vi "Export_mapFileName.vi"(1 "MapFunctionStr":string, 2 "Spectrum":refnum<vi>, 3 "SourceFile":path) -> (0 "Dateipfad":path)   [LabVIEW 2010]
panel:
  in  "Dateiendung":string="tsv"
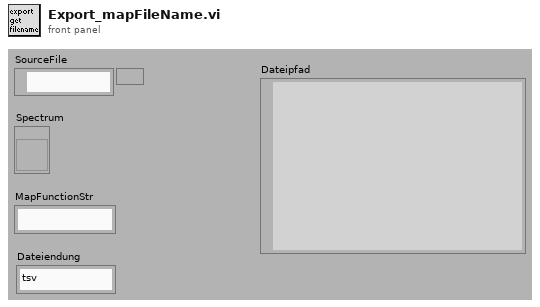
[diagram p1: front panel]
types:
  T1 = typedef "LVCursorListTypeDef.ctl" = cluster{"Name":string, "Color":u32, "Style":u8, "Point Style":u8, "Name Visible":bool, "Allow Drag":bool, "Cursor Mode":u32, "Plot":i32, "Index":i32, "Position":cluster{"X":dbl, "Y":dbl}, "X Scale":u32, "Y Scale":u32, "Watch Plots":i32[], "Watch All Plots":bool, "Plot Area":i32, "Label Offset":cluster{"X":dbl, "Y":dbl}}[]
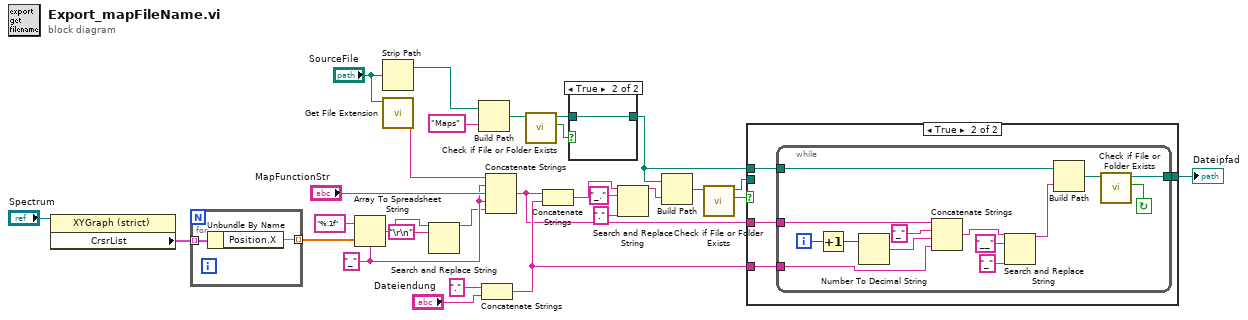
[diagram p0: block diagram]
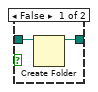
[diagram p2: hidden frame]
diagram:
  w14 = "_" ("String")
  n1 = property on="Eigenschaftsknoten" class="XYGraph (strict)"(reference="Spectrum") -> ("CrsrList"=w20:T1)  [unwired: 1 in, 2 out]
  n2 = for {
    tunnel: w20 -> [w31] mode=indexing
    tunnel: [w30] -> w15 mode=indexing
    n3 = Unbundle By Name(w31) -> ("Position.X"=w30:dbl)
  }
  n4 = Array To Spreadsheet String(delimiter (Tab)=w14, array=w15, 3:"%.1f" ("Format-String")) -> (spreadsheet string=w2:string)
  n5 = Strip Path(path="SourceFile") -> (stripped path=w18:path)  [unwired: 1 out]
  n6 = call <vilib>:"Get File Extension.vi"("file"="SourceFile") -> ("filename without extension"=w17:string)  [unwired: 7 in, 3 out]
  n7 = Search and Replace String(input string=w2, search string="\r\n") -> (result string=w1:string)  [unwired: 6 in, 3 out]
  n8 = Build Path(base path=w18, name or relative path="Maps" ("Name oder relativer Pfad")) -> (appended path=w12:path)
  n9 = Concatenate Strings("." ("String"), "Dateiendung") -> (w24:string)
  n10 = Concatenate Strings(w17, w14, "MapFunctionStr", w14, w1) -> (w19:string)
  n11 = call <vilib>:"Check if File or Folder Exists.vi"("path"=w12) -> ("file or folder exists?"=w11:bool, "dup path"=w10:path)  [unwired: 8 in, 1 out]
  n12 = Concatenate Strings(w19, w24) -> (w6:string)
  n13 = case shown="True" w11 {
    tunnel: w10 -> [w33 w34]
    tunnel: [w32 w34] -> w9
    frame False {
      n14 = Create Folder(path (use dialog)=w33) -> (created path=w32:path)  [unwired: 2 in, 2 out]
    }
    frame True {
    }
  }
  n15 = Search and Replace String(input string=w6, search string="_." ("Such-String"), replace string="." ("String ersetzen(\"\")")) -> (result string=w5:string)  [unwired: 5 in, 3 out]
  n16 = Build Path(base path=w9, name or relative path=w5) -> (appended path=w28:path)
  n17 = call <vilib>:"Check if File or Folder Exists.vi"("path"=w28) -> ("file or folder exists?"=w29:bool, "dup path"=w8:path)  [unwired: 8 in, 1 out]
  n18 = case shown="True" w29 {
    tunnel: [w35 w39] -> w27
    tunnel: w24 -> [_ w38]
    tunnel: w19 -> [_ w37]
    tunnel: w9 -> [_ w36]
    tunnel: w8 -> [w35 _]
    frame False {
    }
    frame True {
      n19 = while {
        tunnel: [w52] -> w39
        tunnel: w38 -> [w40]
        tunnel: w37 -> [w51]
        tunnel: w36 -> [w47]
        i -> [w46]
        stop <- w53 continue-if-true
        n20 = Increment(x=w46) -> (x+1=w45:i32)
        n21 = Number To Decimal String(number=w45) -> (decimal integer string=w50:string)  [unwired: 1 in]
        n22 = Concatenate Strings(w51, "_" ("String"), w50, w40) -> (w44:string)
        n23 = Search and Replace String(input string=w44, search string="__" ("Such-String"), replace string="_" ("String ersetzen(\"\")")) -> (result string=w41:string)  [unwired: 5 in, 3 out]
        n24 = Build Path(base path=w47, name or relative path=w41) -> (appended path=w48:path)
        n25 = call <vilib>:"Check if File or Folder Exists.vi"("path"=w48) -> ("file or folder exists?"=w53:bool, "dup path"=w52:path)  [unwired: 8 in, 1 out]
      }
    }
  }
  "Dateipfad" <- w27
